vi "LaunchMazeUI.vi"   [LabVIEW 2020]
uses:
  App/MazeUI/Main UI.vi
  App/MazeUI/MazeUI.lvclass
panel:
  # "Loading Maze UI..."
types:
  T1 = enum32{"Bad", "Idle", "Run top level", "Running"}
  T2 = enum32{"Invalid", "Standard", "Closed", "Hidden", "Minimized", "Maximized"}
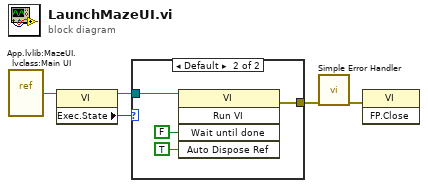
[diagram p0: block diagram]
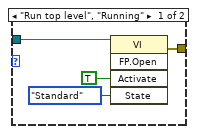
[diagram p2: hidden frame]
diagram:
  n1 = vi-ref "App.lvlib:MazeUI.lvclass:Main UI.vi"() -> (w3:refnum<vi>)
  n2 = property class="VI"(reference=w3) -> (reference out=w1:refnum<vi>, "Exec.State"=w2:T1)  [unwired: 1 in, 1 out]
  n3 = case shown="Default" w2 {
    tunnel: [w6 w12] -> w4
    tunnel: w1 -> [w9 w13]
    frame "Run top level", "Running" {
      n4 = invoke class="VI" method="FP.Open"(reference=w9, "Activate"=TRUE ("Activate?"), "State"=T2."Standard") -> (error out=w6:errorcluster)  [unwired: 2 in, 4 out]
    }
    frame Default {
      n5 = invoke class="VI" method="Run VI"(reference=w13, "Wait until done"=FALSE ("Wait Until Done"), "Auto Dispose Ref"=TRUE ("Auto Dispose Reference")) -> (error out=w12:errorcluster)  [unwired: 2 in, 4 out]
    }
  }
  n6 = call <vilib>:"Simple Error Handler.vi"("error in (no error)"=w4) -> ("error out"=w5:errorcluster)  [unwired: 4 in, 4 out]
  n7 = invoke class="VI" method="FP.Close"(error in=w5) -> ()  [unwired: 2 in, 3 out]
